vi "AB_860_900_Project_RESTfulWebService_Info.vi"(7 "action":T2, 8 "error in (no error)":errorcluster, 10 "RESTfulWebServiceInfo in":T1, 11 "Object In":T3) -> (0 "error out":errorcluster, 2 "RESTfulWebServiceInfo out":T1, 3 "Object Out":T3)   [LabVIEW 2020]
uses:
  <resource>/Framework/Providers/API/ItemRef.ctl
  <vilib>/AppBuilder/RW_Project/AB_RW_Project_PropBag_Action.ctl
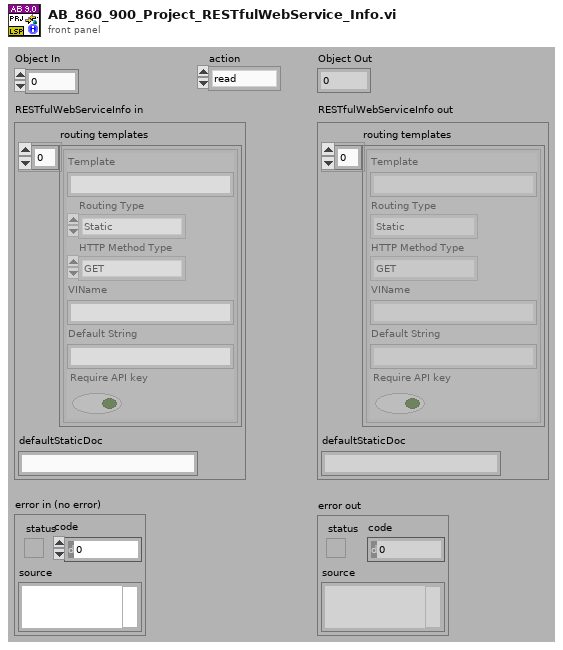
[diagram p1: front panel]
types:
  T1 = cluster{"routing templates":cluster{"Template":string, "Routing Type":enum32{"Method", "Static"}, "HTTP Method Type":enum32{"GET", "POST", "PUT", "DELETE"}, "VIName":string, "Default String":string, "Require API key":bool}[], "defaultStaticDoc":string}
  T2 = typedef "AB_RW_Project_PropBag_Action.ctl" = enum16{"read", "write", "clear", "readPrevious", "writePrevious", "clearPrevious"}
  T3 = typedef "ItemRef.ctl" = u64
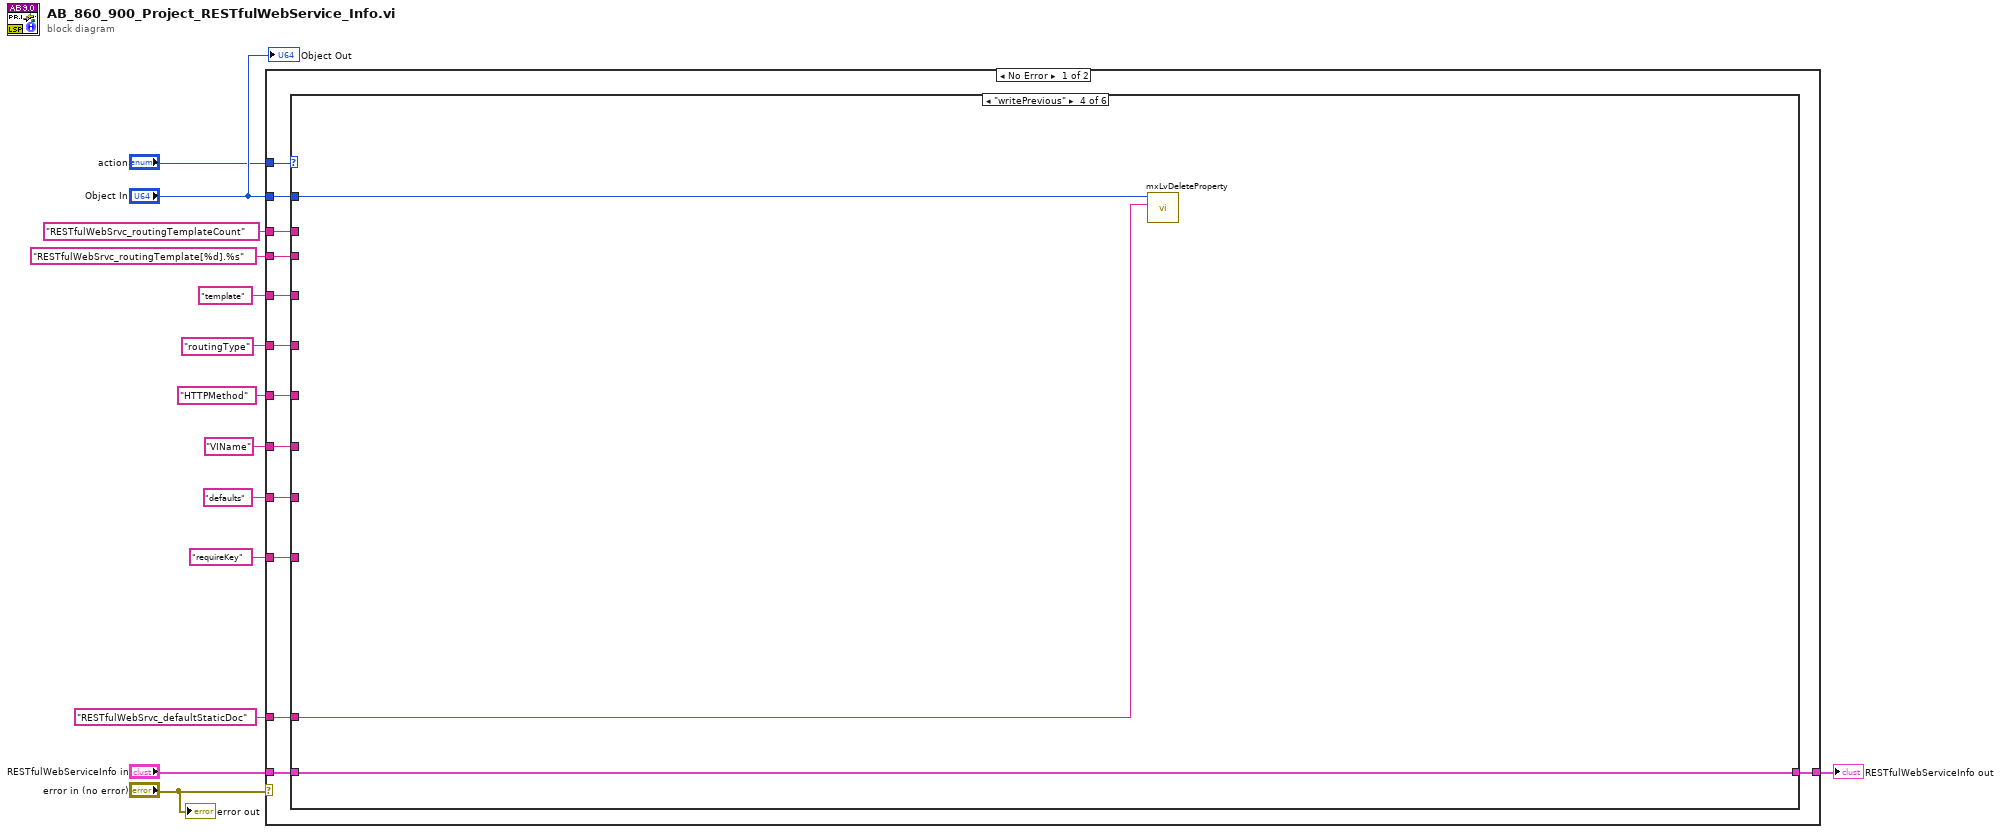
[diagram p0: block diagram]
diagram:
  n1 = case shown="No Error" "error in (no error)" {
    tunnel: "Object In" -> [w27 _]
    tunnel: [w21 _] -> w7
    tunnel: "RESTfulWebSrvc_routingTemplateCount" ("Tag") -> [w26 _]
    tunnel: "RESTfulWebSrvc_routingTemplate[%d].%s" ("Tag") -> [w25 _]
    tunnel: "template" ("Tag") -> [w24 _]
    tunnel: "RESTfulWebServiceInfo in" -> [w23 _]
    tunnel: "action" -> [w22 _]
    tunnel: "routingType" ("Tag") -> [w20 _]
    tunnel: "HTTPMethod" ("Tag") -> [w19 _]
    tunnel: "VIName" ("Tag") -> [w18 _]
    tunnel: "defaults" ("Tag") -> [w17 _]
    tunnel: "requireKey" ("Tag") -> [w16 _]
    tunnel: "RESTfulWebSrvc_defaultStaticDoc" ("Tag") -> [w15 _]
    frame No Error {
      n2 = case shown="\"writePrevious\"" w22 {
        tunnel: w27 -> [_ _ _ w31 _ _]
        tunnel: w26 -> [_ _ _ _ _ _]
        tunnel: w25 -> [_ _ _ _ _ _]
        tunnel: w24 -> [_ _ _ _ _ _]
        tunnel: w23 -> [w28 w29 w30 w33 w34 w35]
        tunnel: [w28 w29 w30 w33 w34 w35] -> w21
        tunnel: w20 -> [_ _ _ _ _ _]
        tunnel: w19 -> [_ _ _ _ _ _]
        tunnel: w18 -> [_ _ _ _ _ _]
        tunnel: w17 -> [_ _ _ _ _ _]
        tunnel: w16 -> [_ _ _ _ _ _]
        tunnel: w15 -> [_ _ _ w32 _ _]
        frame "read" {
        }
        frame "write" {
        }
        frame "clear" {
        }
        frame "writePrevious" {
          n3 = call <resource>:"mxLvDeleteProperty.vi"("Tag"=w32, "Item"=w31) -> ()  [unwired: 1 in, 9 out]
        }
        frame "readPrevious" {
        }
        frame "clearPrevious" {
        }
      }
    }
    frame Error {
    }
  }
  "RESTfulWebServiceInfo out" <- w7
  "Object Out" <- "Object In"
  "error out" <- "error in (no error)"
